vi "TCPReceiveComparer.vi"(10 "Compare String":string, 11 "Recieved String":string) -> (3 "Match":bool)   [LabVIEW 2017]
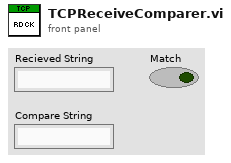
[diagram p1: front panel]
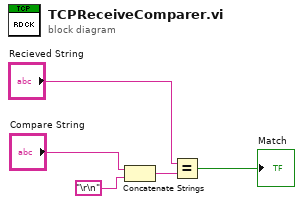
[diagram p0: block diagram]
diagram:
  n1 = Concatenate Strings("Compare String", "\r\n") -> (w2:string)
  n2 = Equal?(x="Recieved String", y=w2) -> (x = y?=→"Match":bool)
